vi "Write Limit Test Type.vi"(8 "error in (no error)":errorcluster, 10 "Limit Test Type":T1, 11 "Test Numeric in":refnum<class "Test Numeric.lvclass">) -> (0 "error out":errorcluster, 3 "Test Numeric out":refnum<class "Test Numeric.lvclass">)   [LabVIEW 2021, in "BT.lvlib" / "Test Numeric.lvclass"]
uses:
  Test Numeric.lvclass
  Test Numeric.lvclass/Test Numeric.ctl
  Support/Limit Test Type.ctl
  BT.lvlib
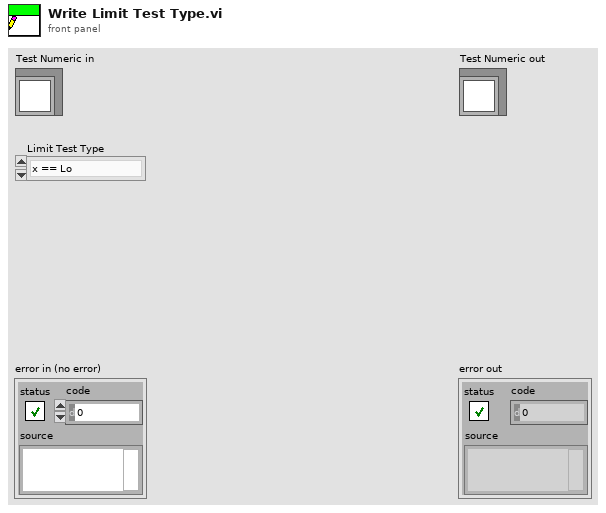
[diagram p1: front panel]
types:
  T1 = typedef "BT.lvlib/Limit Test Type.ctl" = enum16{"x == Lo", "x != Lo", "x > Lo", "x < Lo", "x >= Lo", "x <= Lo", "Lo > x < Hi", "Lo >= x <= Hi", "Lo >= x < Hi", "Lo > x <= Hi", "Lo < x > Hi", "Lo <= x >= Hi", "Lo <= x > Hi", "Lo < x >= Hi", "x == Lo +/- Hi"}
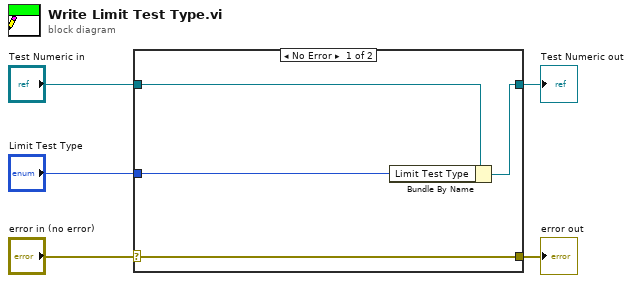
[diagram p0: block diagram]
diagram:
  n1 = case shown="No Error" "error in (no error)" {
    selector: "error in (no error)" -> [w9 w10]
    tunnel: [w9 w10] -> w4
    tunnel: [w7 w11] -> w2
    tunnel: "Test Numeric in" -> [w8 w11]
    tunnel: "Limit Test Type" -> [w6 _]
    frame No Error {
      n2 = Bundle By Name(cluster=w8, "Limit Test Type"=w6) -> (w7:refnum<class "Test Numeric.lvclass">)
    }
    frame Error {
    }
  }
  "error out" <- w4
  "Test Numeric out" <- w2
